vi "programacion 9 parcial 2.vi"() -> ()   [LabVIEW 2011]
panel:
  in  "salir":bool
  in  "Sumar columnas":bool
  in  "Rellenar":bool
  out "Array":dbl[][](array[numeric])
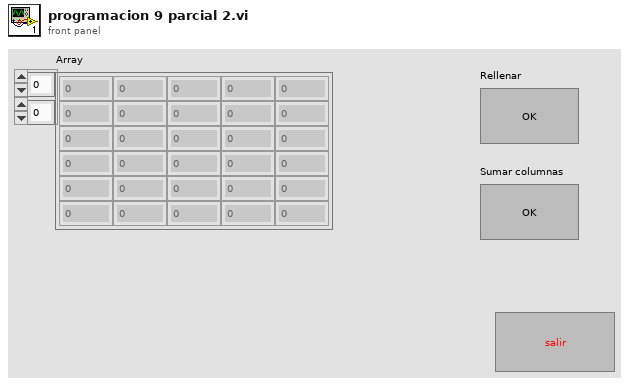
[diagram p1: front panel]
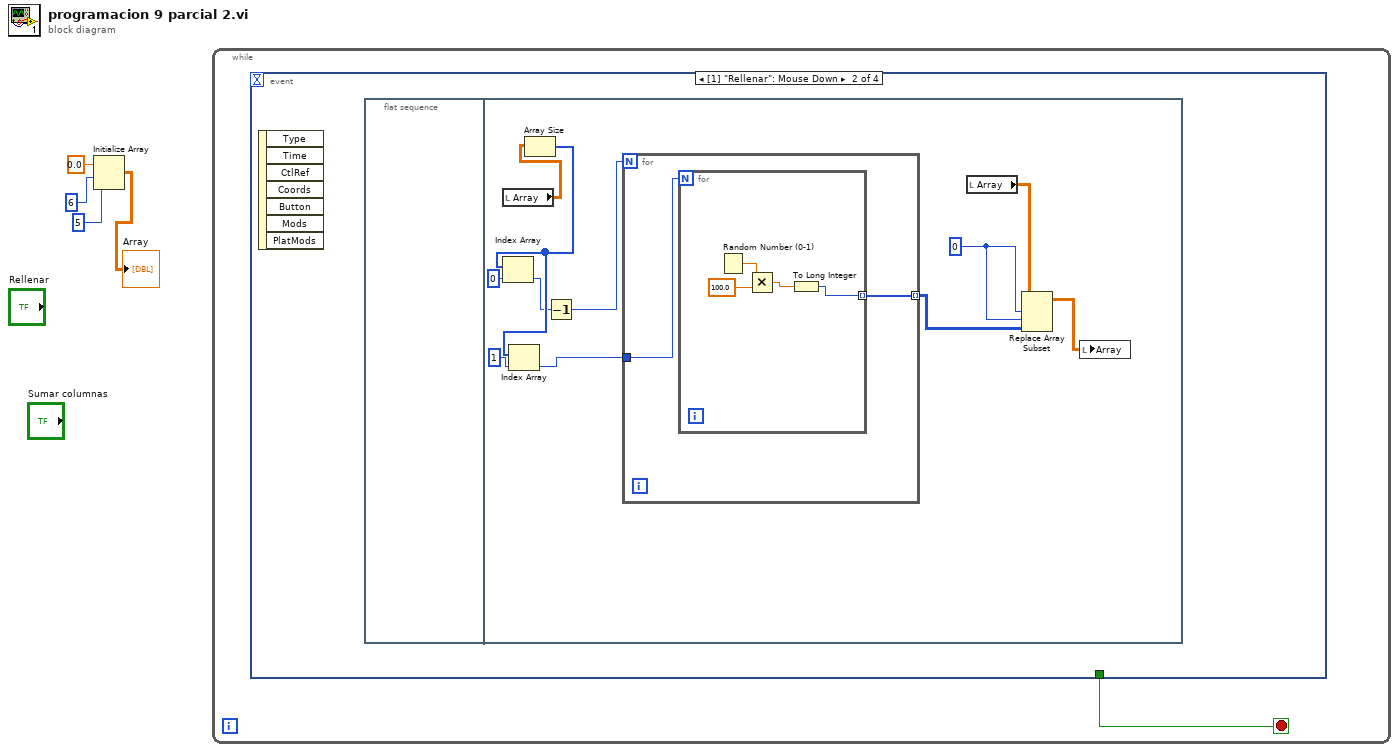
[diagram p0: block diagram]
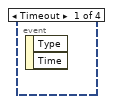
[diagram p2: hidden frame]
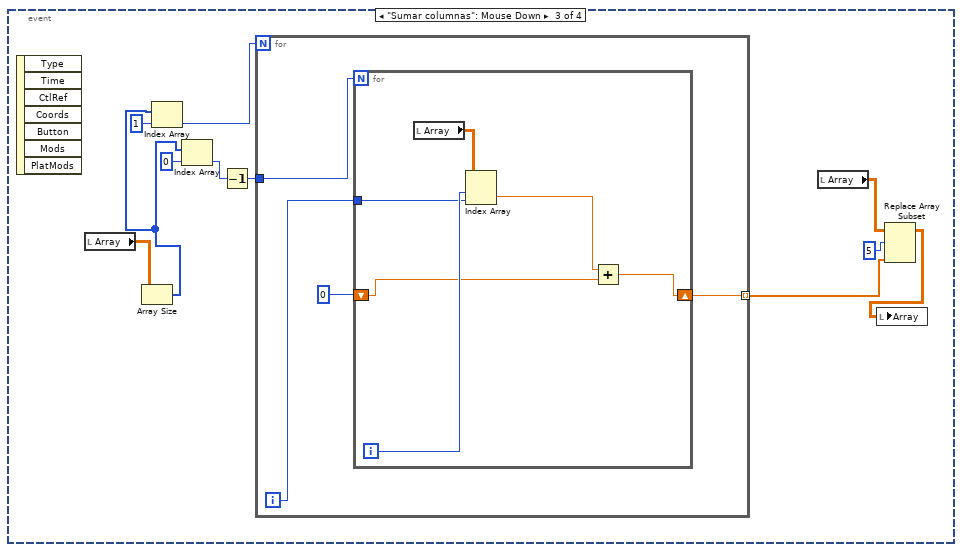
[diagram p3: hidden frame]
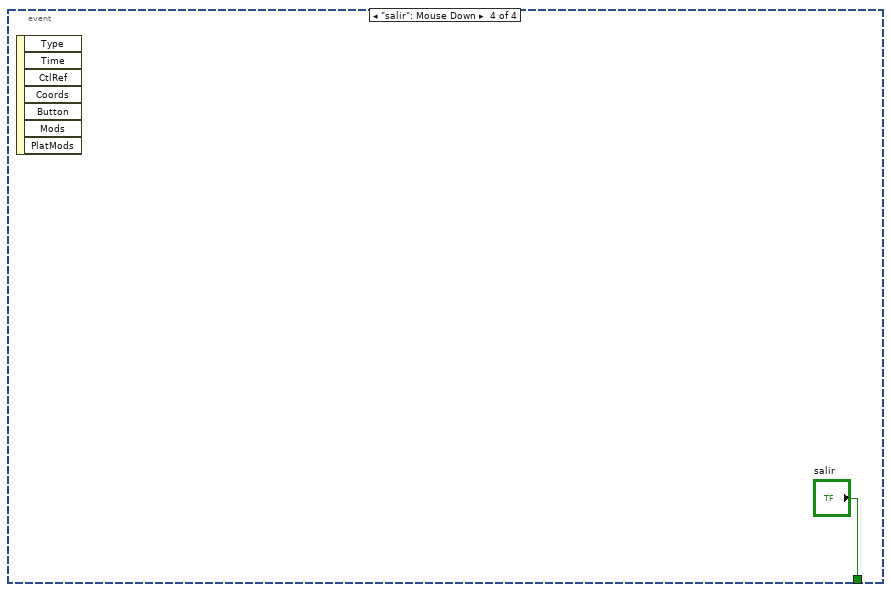
[diagram p4: hidden frame]
diagram:
  n1 = Initialize Array "Initialize Array"(0.0 ("element"), 6 ("dimension size"), 5 ("dimension size")) -> (→"Array":dbl[][])
  n2 = while {
    stop <- w5 stop-if-true
    n3 = event shown="[1] \"Rellenar\": Mouse Down" {
      selector: _ -> [_ _ _ _]
      dyn-events: _ -> [_ _ _ _]
      timeout: _ -> [_ _ _ _]
      tunnel: [_ _ _ "salir"] -> w5
      event Timeout {
        n4 = event-data() -> ()  [unwired: 1 in, 2 out]
      }
      event "Rellenar": Mouse Down {
        n5 = event-data() -> ()  [unwired: 1 in, 7 out]
        n6 = flat-sequence {
          frame #0 {
          }
          frame #1 {
            w8 = 0
            n7 = local read "Array"() -> (w16:dbl[][])
            n8 = Array Size(array=w16) -> (size(s)=w14:i32[])
            n9 = Index Array "Index Array"(array=w14, index=0) -> (element=w11:i32)
            n10 = Index Array "Index Array"(array=w14, index=1) -> (element=w12:i32)
            n11 = Decrement(x=w11) -> (x-1=w10:i32)
            n12 = for {
              N: w10 -> [_]
              tunnel: w12 -> [w18]
              tunnel: [w17] -> w7 mode=indexing
              n13 = for {
                N: w18 -> [_]
                tunnel: [w19] -> w17 mode=indexing
                n14 = Random Number (0-1)() -> (number: 0 to 1=w22:dbl)
                n15 = Multiply(x=w22, y=100.0) -> (x*y=w20:dbl)
                n16 = To Long Integer(number=w20) -> (32bit integer=w19:i32)
              }
            }
            n17 = local read "Array"() -> (w9:dbl[][])
            n18 = Replace Array Subset(array=w9, new element=w7, index (row)=w8, index (col)=w8) -> (w6:dbl[][])
            n19 = local write "Array"(w6) -> ()
          }
        }
      }
      event "Sumar columnas": Mouse Down {
        n20 = event-data() -> ()  [unwired: 1 in, 7 out]
        n21 = local read "Array"() -> (w33:dbl[][])
        n22 = Array Size(array=w33) -> (size(s)=w24:i32[])
        n23 = Index Array "Index Array"(array=w24, index=1) -> (element=w32:i32)
        n24 = Index Array "Index Array"(array=w24, index=0) -> (element=w30:i32)
        n25 = Decrement(x=w30) -> (x-1=w28:i32)
        n26 = for {
          N: w32 -> [_]
          tunnel: w28 -> [w37]
          tunnel: [w34] -> w26 mode=indexing
          i -> [w36]
          n27 = for {
            N: w37 -> [_]
            tunnel: w36 -> [w42]
            shift-right: [w39] -> w34
            shift-left: 0 -> [w40]
            i -> [w43]
            n28 = local read "Array"() -> (w38:dbl[][])
            n29 = Index Array(array=w38, index (row)=w43, index (col)=w42) -> (element=w41:dbl)
            n30 = Add(x=w41, y=w40) -> (x+y=w39:dbl)
          }
        }
        n31 = local read "Array"() -> (w27:dbl[][])
        n32 = Replace Array Subset "Replace Array Subset"(array=w27, new element=w26, index (row)=5 ("disabled index (col)")) -> (w25:dbl[][])  [unwired: 1 in]
        n33 = local write "Array"(w25) -> ()
      }
      event "salir": Mouse Down {
        n34 = event-data() -> ()  [unwired: 1 in, 7 out]
      }
    }
  }
